vi "add Test.vi"(8 "error in (no error)":errorcluster caption="Fehler (Eingang, kein Fehler)", 10 "Test.lvclass":refnum<class "Test.lvclass">, 11 "Test Eingang":refnum<class "Norm.lvclass"> caption="Norm in") -> (0 "error out":errorcluster caption="Fehler (Ausgang)", 3 "Test Ausgang":refnum<class "Norm.lvclass"> caption="Norm out")   [LabVIEW 2013, in "DatenKlassen.lvlib" / "Norm.lvclass"]
uses:
  Norm.lvclass
  Test/Test.lvclass
  Norm.lvclass/Norm.ctl
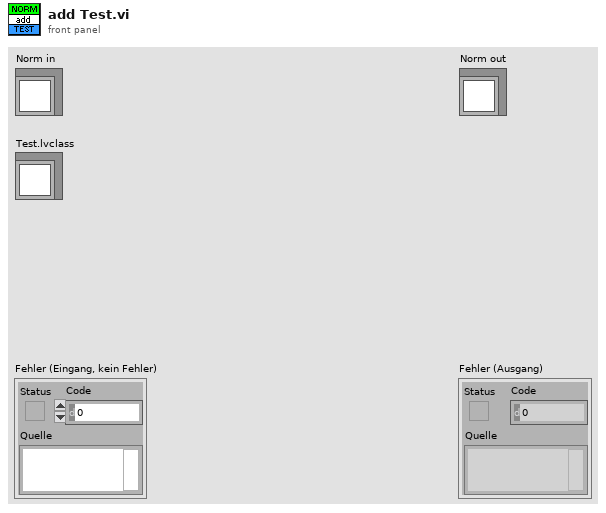
[diagram p1: front panel]
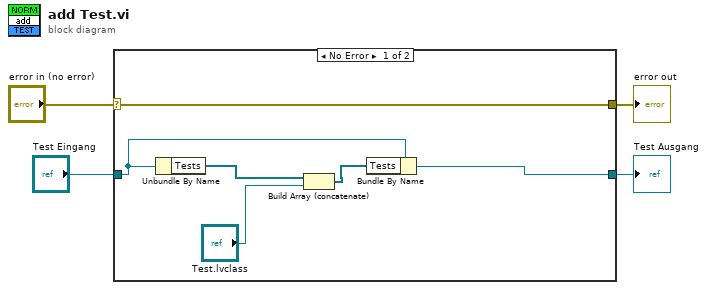
[diagram p0: block diagram]
diagram:
  n1 = case shown="No Error" "error in (no error)" {
    selector: "error in (no error)" -> [w10 w12]
    tunnel: [w10 w12] -> w3
    tunnel: [w8 w11] -> w1
    tunnel: "Test Eingang" -> [w9 w11]
    frame No Error {
      n2 = Unbundle By Name(w9) -> ("Tests"=w7:refnum<class "Test.lvclass">[])
      n3 = Build Array (concatenate)(w7, "Test.lvclass") -> (w5:refnum<class "Test.lvclass">[])
      n4 = Bundle By Name(cluster=w9, "Tests"=w5) -> (w8:refnum<class "Norm.lvclass">)
    }
    frame Error {
    }
  }
  "error out" <- w3
  "Test Ausgang" <- w1
